vi "Stop Core.vi"(10 "final error code":i32, 11 "Caller in":refnum<class "Actor.lvclass">) -> (3 "Caller out":refnum<class "Actor.lvclass">)   [LabVIEW 2020, in "Actor.lvlib" / "Actor.lvclass"]
doc: "(<B>Filename</B>: Actor Framework.lvlib:Actor.lvclass:Stop Core.vi)\n\nDefines what the actor does before it stops. Use the <B>final error code</B> input to determine whether the actor shut down in response to an error.\n\nBy default, this method passes the Stop message along to all auto-stop nested actors. A descendant class may override this method to define additional behavior, such as shutting down any processes the actor initiated in its override of the Actor Core method."
uses:
  Actor.lvclass
  Actor.lvclass/Actor.ctl
  <vilib>/ActorFramework/Actor/Actor.lvclass
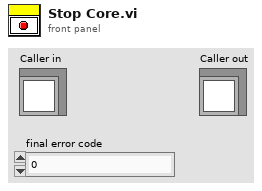
[diagram p1: front panel]
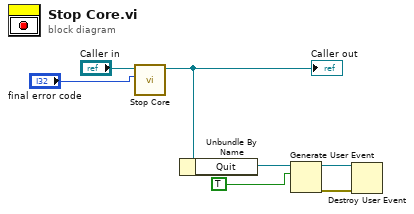
[diagram p0: block diagram]
diagram:
  n1 = call-parent "Stop Core.vi"("final error code"="final error code", "Actor in"="Caller in") -> ("Actor out"=w5:refnum<class "Actor.lvclass">)  [unwired: 9 in]
  "Caller out" <- w5
  n2 = Unbundle By Name(w5) -> ("Quit"=w4:refnum<user-event>)
  n3 = Generate User Event(user event=w4, event data cluster=TRUE) -> (user event out=w2:refnum<user-event>, error out=w1:errorcluster)  [unwired: 2 in]
  n4 = Destroy User Event(user event=w2, error in=w1) -> ()  [unwired: 1 out]
